vi "set fractional flows.vi"(0 "State Settings":T6[][](array[typedef]) {"valve cycle time" min=0.2 step=0.1 format="%.2f"; "flow division"."5" min=0.0 max=1.0 step=0.01 format="%.3f"; "flow division"."4" min=0.0 max=1.0 step=0.01 format="%.3f"; "flow division"."3" min=0.0 max=1.0 step=0.01 format="%.3f"; "flow division"."2" min=0.0 max=1.0 step=0.01 format="%.3f"; "flow division"."1" min=0.0 max=1.0 step=0.01 format="%.3f"; "flow rate" format="%.3f"}, 1 "Index Values":u32[](array[numeric]), 3 "Method settings":T2 {"Column"."porosity" format="%.4f"; "Column"."diameter" format="%.2f"; "Column"."length" format="%.2f"}) -> (5 "Control Settings":T4 {"Pump speed" format="%.2f"}, 6 "State Settings out":T6[][](array[typedef]) {"valve cycle time" min=0.2 step=0.1 format="%.2f"; "flow division"."5" min=0.0 max=1.0 step=0.01 format="%.3f"; "flow division"."4" min=0.0 max=1.0 step=0.01 format="%.3f"; "flow division"."3" min=0.0 max=1.0 step=0.01 format="%.3f"; "flow division"."2" min=0.0 max=1.0 step=0.01 format="%.3f"; "flow division"."1" min=0.0 max=1.0 step=0.01 format="%.3f"; "flow rate" format="%.3f"}, 7 "column flow":T1 {"t/q" format="%.3f"; "Velocity" format="%.3f"}, 8 "toggle valves":bool[](array[boolean]), 9 "show fractions":bool)   [LabVIEW 2012]
uses:
  Peristaltic/pump rpm poly.vi/pump control.vi
  State Setting.ctl
  Stamp/Switch settings vertical.ctl
  flow fraction.ctl
  Peristaltic/3-stop colors.ctl
  Stamp/Stamp Controls.ctl
  Method settings.ctl
  column flow.ctl
  switches.ctl
panel:
  # "rpm"
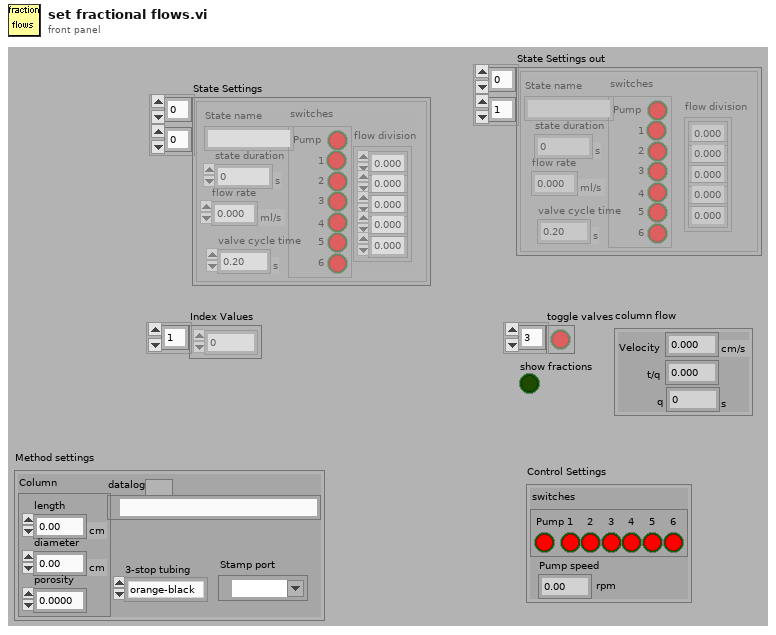
[diagram p1: front panel]
types:
  T1 = typedef "column flow.ctl" = cluster{"Velocity":dbl[unit], "t/q":dbl, "q":dbl[unit]}
  T2 = typedef "Method settings.ctl" = cluster{"3-stop tubing":T3, "Stamp port":refnum<visa-resource-name>, "datalog":path, "Column":cluster{"length":dbl[unit], "diameter":dbl[unit], "porosity":dbl}}
  T3 = typedef "3-stop colors.ctl" = enum16{"orange-black", "orange-red", "orange-blue", "orange-green", "green-yellow", "orange-yellow", "white-yellow", "orange-white", "black-black", "orange-orange", "white-black", "white-white", "white-red", "red-red", "red-grey", "grey-grey", "yellow-yellow", "yellow-blue", "blue-blue", "blue-green", "green-green", "purple-purple", "purple-black", "purple-orange", "purple-white", "black-white", "13", "14", "15", "16", "17", "18"}
  T4 = typedef "Stamp Controls.ctl" = cluster{"Pump speed":dbl, "switches":T5}
  T5 = typedef "switches.ctl" = cluster{"Pump":bool, "1":bool, "2":bool, "3":bool, "4":bool, "5":bool, "6":bool}
  T6 = typedef "State Setting.ctl" = cluster{"switches":T7, "flow rate":dbl[unit], "flow division":cluster{"1":T8, "2":T8, "3":T8, "4":T8, "5":T8}, "State name":string, "state duration":dbl[unit], "valve cycle time":dbl[unit]}
  T7 = typedef "Switch settings vertical.ctl" = cluster{"Pump":bool, "1":bool, "2":bool, "3":bool, "4":bool, "5":bool, "6":bool}
  T8 = typedef "flow fraction.ctl" = dbl
  T9 = cluster{"[0]":T8, "[1]":T8, "[2]":T8, "[3]":T8, "[4]":T8}
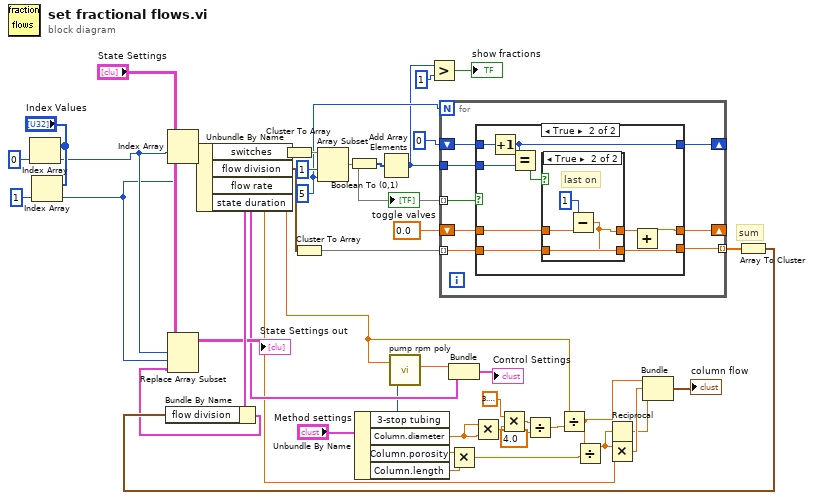
[diagram p0: block diagram]
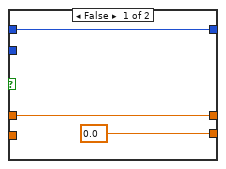
[diagram p2: hidden frame]
diagram:
  w39 = 5 ("length")
  # "sum"
  n1 = Index Array(array="Index Values", index=0) -> (element=w18:u32)
  n2 = Index Array(array="Index Values", index=1) -> (element=w17:u32)
  n3 = Index Array(array="State Settings", index (row)=w18, index (col)=w17) -> (element=w40:T6)
  n4 = Unbundle By Name(w40) -> ("switches"=w25:T7, "flow division"=w38:cluster{"1":T8, "2":T8, "3":T8, "4":T8, "5":T8}, "flow rate"=w11:dbl[unit], "state duration"=w4:dbl[unit])
  n5 = Cluster To Array(cluster=w25) -> (array=w41:bool[])
  n6 = Cluster To Array(cluster=w38) -> (array=w35:T8[])
  n7 = Array Subset(array=w41, index=1, length=w39) -> (w43:bool[])
  "toggle valves" <- w43
  n8 = Boolean To (0,1)(Boolean=w43) -> (0, 1=w44:i16[])
  n9 = Unbundle By Name("Method settings") -> ("3-stop tubing"=w22:T3, "Column.diameter"=w16:dbl[unit], "Column.porosity"=w6:dbl, "Column.length"=w9:dbl[unit])
  n10 = Add Array Elements(numeric array=w44) -> (sum=w29:i16)
  n11 = call-poly "pump rpm poly.vi"(0:w11, 1:w22) -> ("pump speed (rpm)"=w26:dbl)  [unwired: 2 in, 1 out]
  n12 = Greater?(x=w29, y=i16 1) -> (0:→"show fractions":bool)
  n13 = for {
    N: w39 -> [_]
    shift-right: [w49] -> _
    shift-left: i16 0 ("y") -> [w51]
    tunnel: w43 -> [w52] mode=indexing
    tunnel: w29 -> [w50]
    shift-right: [w48] -> _
    shift-left: 0.0 ("y") -> [w47]
    tunnel: [w46] -> w34 mode=indexing
    tunnel: w35 -> [w45] mode=indexing
    n14 = case shown="True" w52 {
      tunnel: w51 -> [w55 w64]
      tunnel: w50 -> [_ w63]
      tunnel: [w55 w62] -> w49
      tunnel: [w54 w57] -> w48
      tunnel: w47 -> [w54 w56]
      tunnel: [0.0 ("y") w60] -> w46
      tunnel: w45 -> [_ w59]
      frame False {
      }
      frame True {
        n15 = Increment(x=w64) -> (x+1=w62:i16)
        n16 = Equal?(x=w62, y=w63) -> (x = y?=w61:bool)
        n17 = case shown="True" w61 {
          tunnel: [w66 w67] -> w58
          tunnel: w56 -> [w66 w69]
          tunnel: [w65 w67] -> w60
          tunnel: w59 -> [w65 _]
          frame False {
          }
          frame True {
            # "last on"
            n18 = Subtract(x=1, y=w69) -> (x-y=w67:T8)
          }
        }
        n19 = Add(x=w58, y=w59) -> (x+y=w57:T8)
      }
    }
  }
  n20 = Bundle("pump speed (rpm)"=w26, "switches"=w25) -> (→"Control Settings":cluster{"pump speed (rpm)":dbl, "switches":T7})  [unwired: 1 in]
  n21 = Multiply(x=w6, y=w9) -> (x*y=w5:dbl[unit])
  n22 = Multiply(x=w16, y=w16) -> (x*y=w15:dbl[unit])
  n23 = Multiply(x=3.141592653589793, y=w15) -> (x*y=w13:dbl[unit])
  n24 = Divide(x=w13, y=4.0) -> (x/y=w8:dbl[unit])
  n25 = Divide(x=w11, y=w8) -> (x/y=w7:dbl[unit])
  n26 = Divide(x=w7, y=w5) -> (x/y=w2:dbl[unit])
  n27 = Reciprocal(x=w2) -> (1/x=w1:dbl[unit])
  n28 = Multiply(x=w2, y=w4) -> (x*y=w3:dbl)
  n29 = Bundle(w7, w3, w1) -> (→"column flow":cluster{dbl[unit], dbl, dbl[unit]})  [unwired: 1 in]
  n30 = Array To Cluster(array=w34) -> (cluster=w33:T9)
  n31 = Bundle By Name(cluster=w40, "flow division"=w33) -> (w32:T6)
  n32 = Replace Array Subset(array="State Settings", new element=w32, index (row)=w18, index (col)=w17) -> (→"State Settings out":T6[][])
